vi "testUintArrayMaxMin.vi"(8 "error in (no error)":errorcluster, 11 "TestCase in":refnum<class "UnitTestUintClass.lvclass">) -> (0 "error out":errorcluster, 3 "TestCase out":refnum<class "UnitTestUintClass.lvclass">)   [LabVIEW 2011, in "UnitTestUintClass.lvclass"]
uses:
  UnitTestUintClass.lvclass
  UnitTestUintClass.lvclass/UnitTestUintClass.ctl
  <vilib>/addons/_JKI Toolkits/VI Tester/TestCase.llb/TestCase.lvclass
  UintClass/UintClass.lvclass
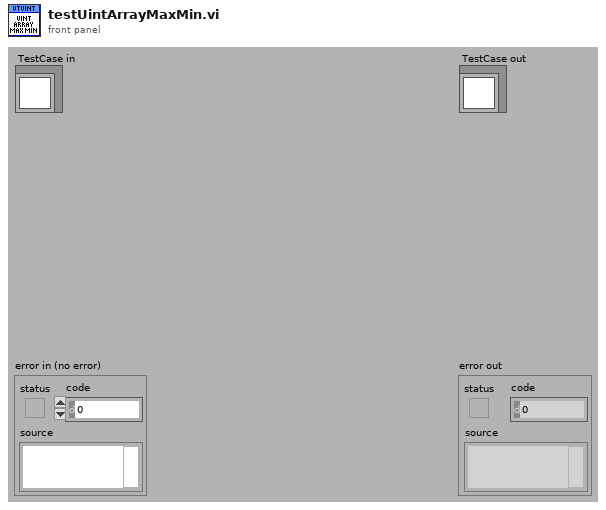
[diagram p1: front panel]
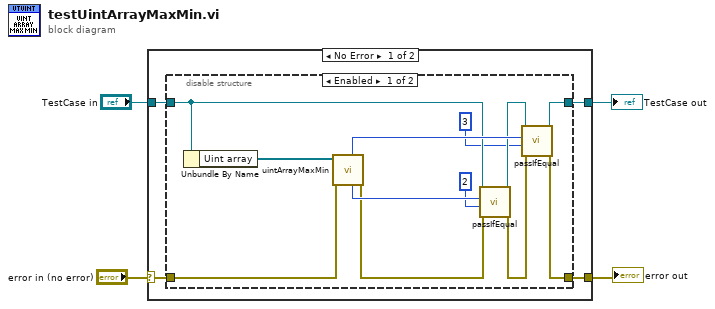
[diagram p0: block diagram]
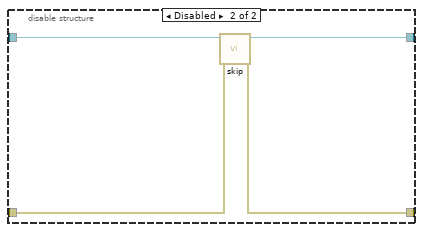
[diagram p2: hidden frame]
diagram:
  n1 = case shown="No Error" "error in (no error)" {
    selector: "error in (no error)" -> [w6 w26]
    tunnel: [w5 w26] -> w3
    tunnel: [w7 w25] -> w1
    tunnel: "TestCase in" -> [w8 w25]
    frame No Error {
      n2 = disable-structure shown="Enabled" {
        disable-tunnel: w8 -> [w13 w24]
        disable-tunnel: [w20 w21] -> w7
        disable-tunnel: w6 -> [w18 w23]
        disable-tunnel: [w19 w22] -> w5
        frame Enabled {
          n3 = Unbundle By Name(w13) -> ("Uint array"=w17:refnum<class "UintClass.lvclass">[])
          n4 = call "uintArrayMaxMin.vi"("Error in (no error)"=w18, "Uint array in"=w17) -> ("Error out"=w12:errorcluster, "Index min"=w15:i32, "Index max"=w16:i32)  [unwired: 4 in, 3 out]
          n5 = call-dynamic "passIfEqual.vi"("error in (no error)"=w12, "y"=2 ("Index min"), "x"=w15, "TestCase in"=w13) -> ("error out"=w11:errorcluster, "TestCase out"=w14:refnum<class "UnitTestUintClass.lvclass">)  [unwired: 6 in]
          n6 = call-dynamic "passIfEqual.vi"("error in (no error)"=w11, "y"=3 ("Index min"), "x"=w16, "TestCase in"=w14) -> ("error out"=w19:errorcluster, "TestCase out"=w20:refnum<class "UnitTestUintClass.lvclass">)  [unwired: 6 in]
        }
        frame Disabled {
          n7 = call <vilib>:"skip.vi"("error in (no error)"=w23, "TestCase in"=w24) -> ("error out"=w22:errorcluster, "TestCase out"=w21:refnum<class "UnitTestUintClass.lvclass">)  [unwired: 8 in]
        }
      }
    }
    frame Error {
    }
  }
  "error out" <- w3
  "TestCase out" <- w1
